vi "Set VI Separate Compiled Code.vi"() -> ()   [LabVIEW 2016]
doc: "A wrapper engine for setting separate compiled code for all VIs in a folder."
uses:
  <vilib>/Utility/error.llb/DialogType.ctl
  SLL Queued State Machine/Queue Driver/Create Queue.vi
  SLL Queued State Machine/Queue Driver/Enqueue an Item to Queue.vi
  SLL Queued State Machine/Queue Driver/Dequeue Queue.vi
  SLL Queued State Machine/Queue Driver/Enqueue N Items.vi
  SLL Queued State Machine/Queue Driver/Flush Queue.vi
  SLL Queued State Machine/Queue Driver/Release Queue.vi
  SLL Queued State Machine/SLL QSM.lvlib
panel:
  out "Progress":i32
  in  "Separate Compiled Code?":bool=TRUE
  out "VI List[]":path[](array[path])
  in  "Folder Path":path
  out "Status":string
  in  "Run":bool
  # "Set VI Separate Compiled Code"
  # "Sets the separate compile code property for the VIs in the folder"
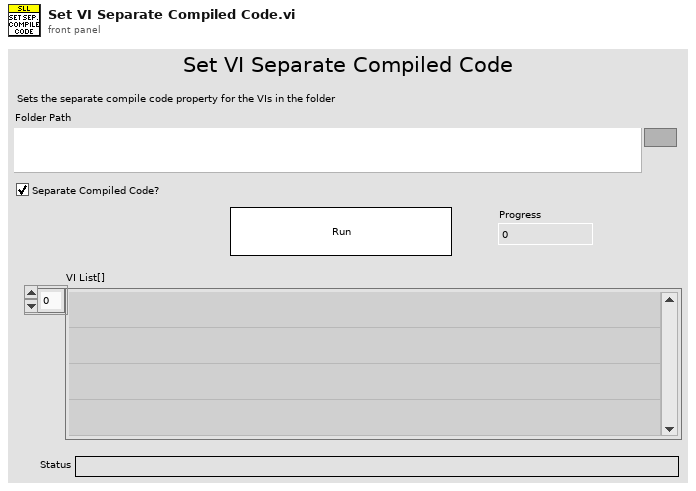
[diagram p1: front panel]
types:
  T1 = typedef "DialogType.ctl" = u16
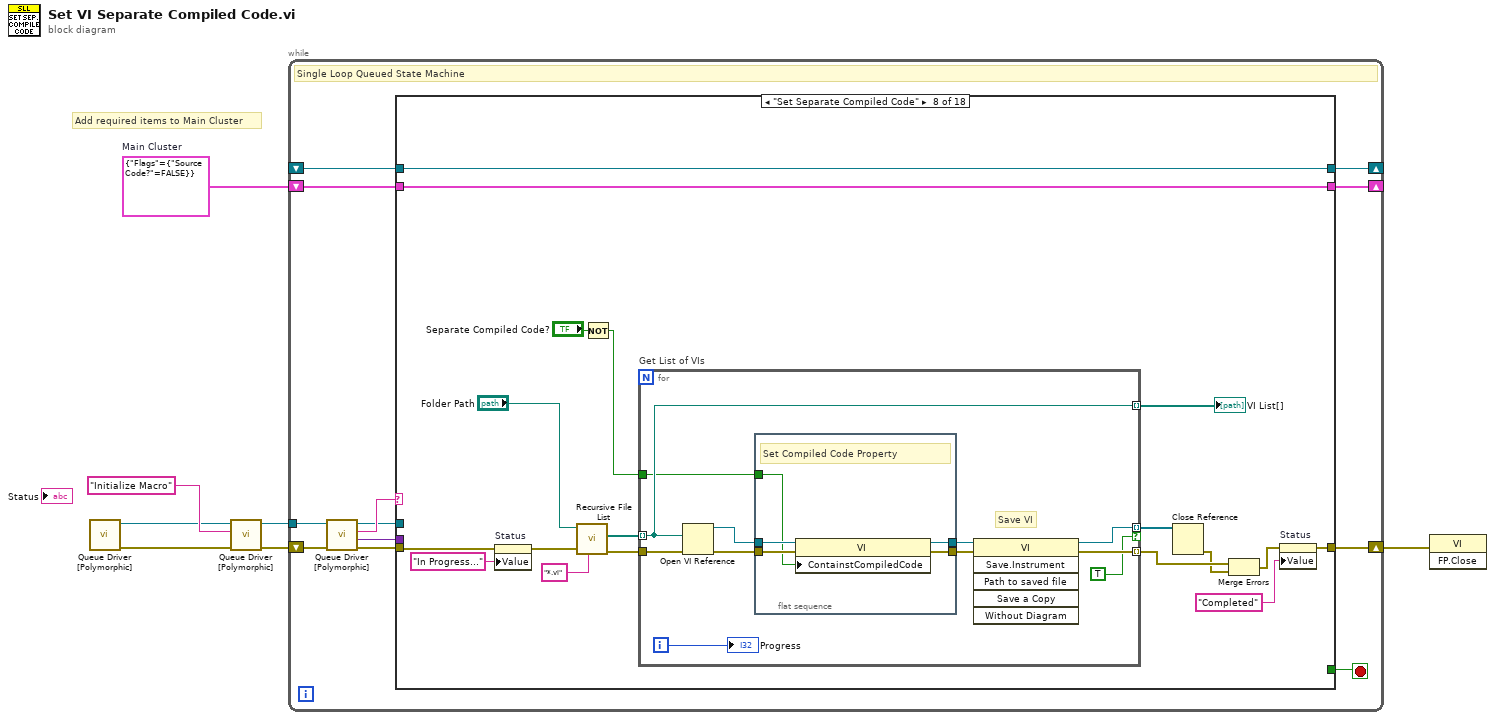
[diagram p0: block diagram]
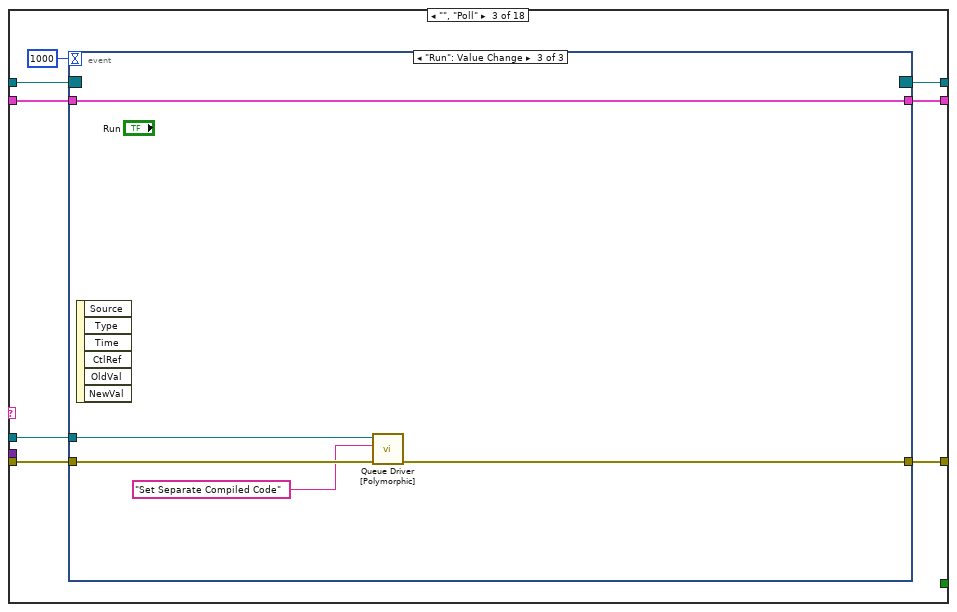
[diagram p4: hidden frame]
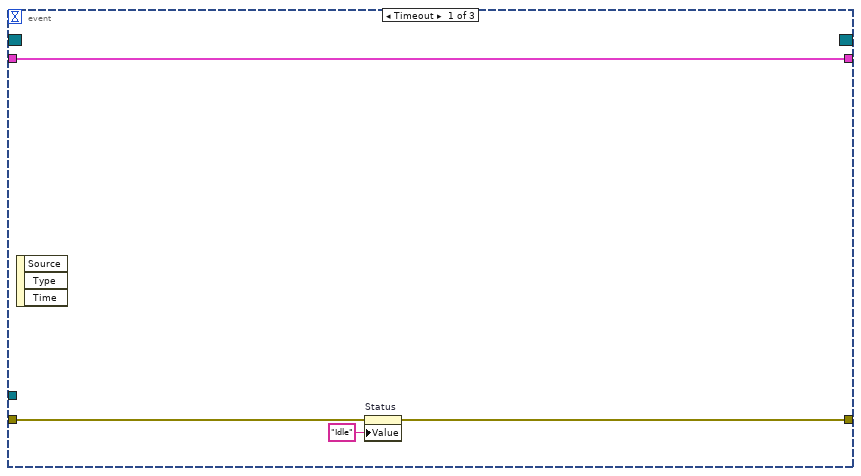
[diagram p5: hidden frame]
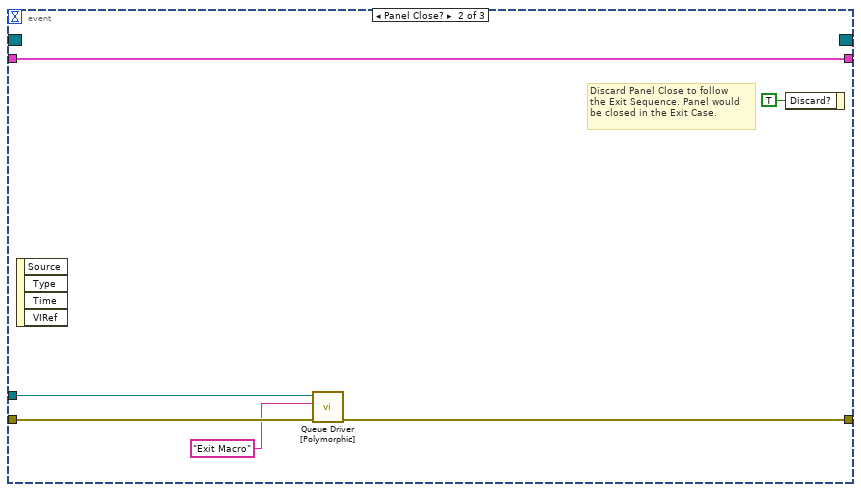
[diagram p6: hidden frame]
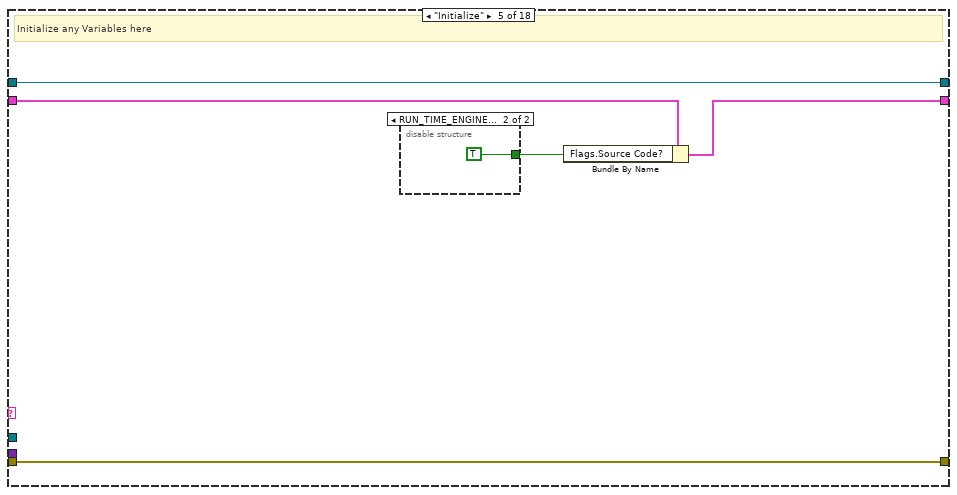
[diagram p8: hidden frame]
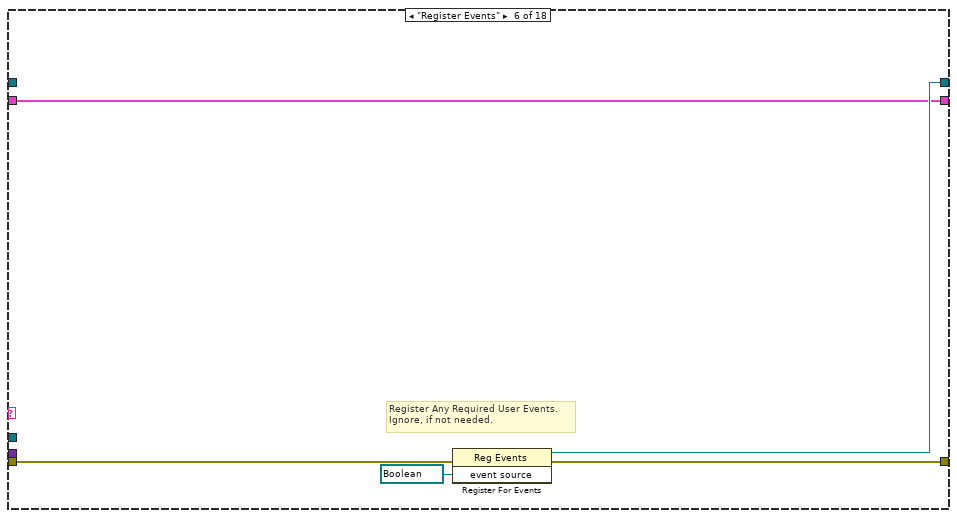
[diagram p10: hidden frame]
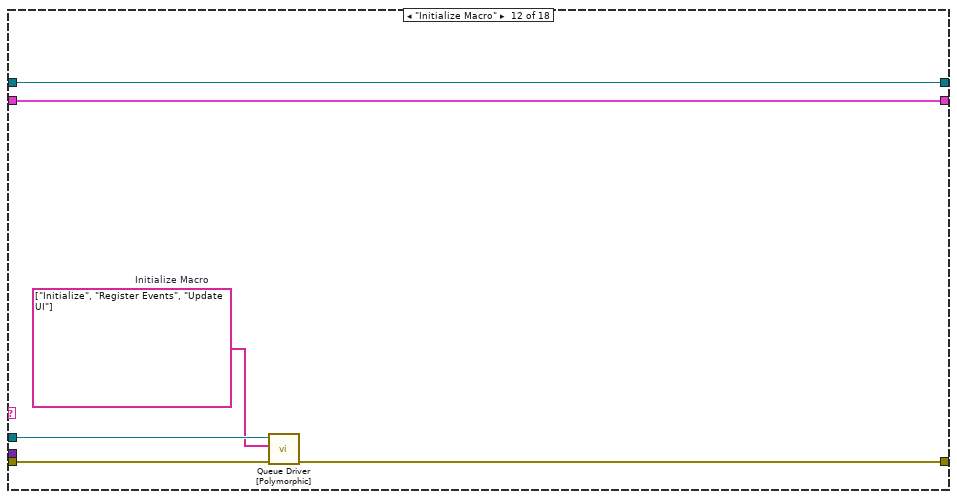
[diagram p15: hidden frame]
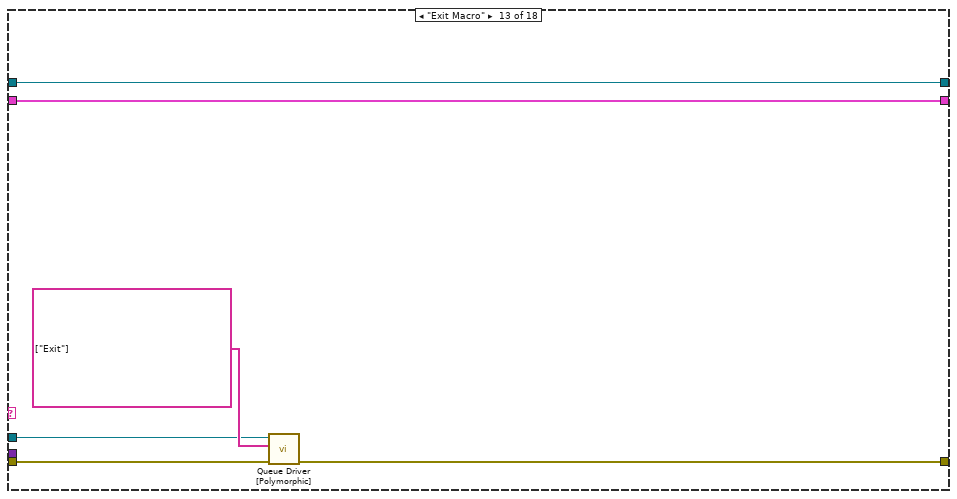
[diagram p16: hidden frame]
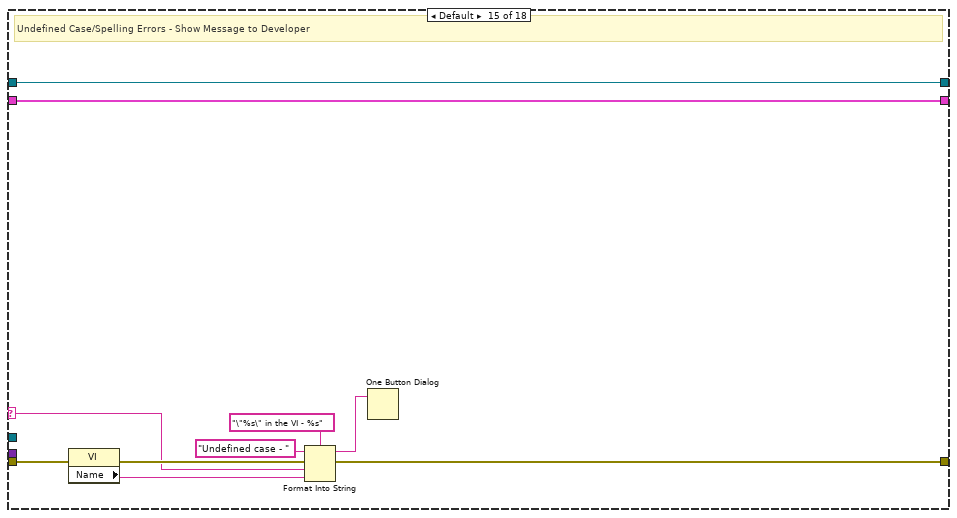
[diagram p18: hidden frame]
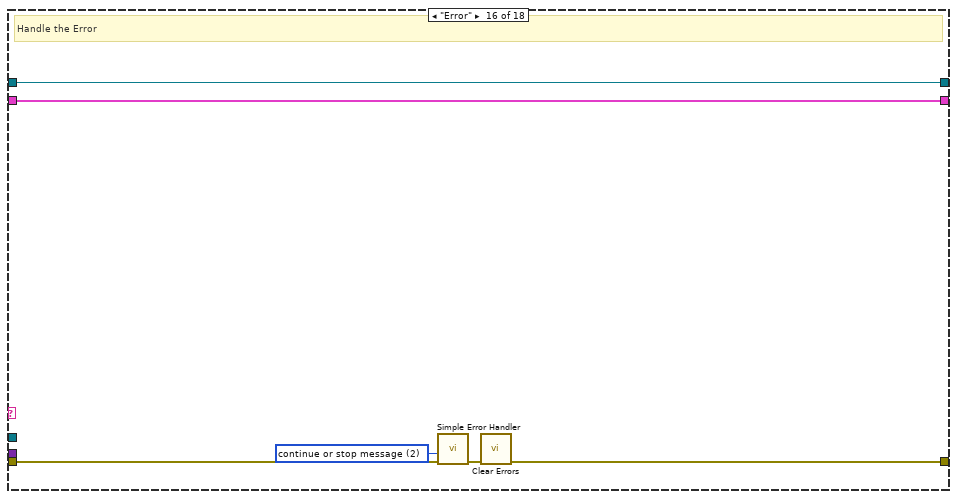
[diagram p19: hidden frame]
diagram:
  w5 = cluster{"Flags":cluster{"Source Code?":bool}} {"Flags"={"Source Code?"=FALSE}}  # Main Cluster
  # "Add required items to Main Cluster"
  n1 = call-poly "Queue Driver [Polymorphic].vi"() -> ("Error Out"=w7:errorcluster, "Queue Ref"=w3:refnum<queue>)  [unwired: 10 in]
  n2 = call-poly "Queue Driver [Polymorphic].vi"("Error In"=w7, "Item to Add"="Initialize Macro", "Queue Ref In"=w3) -> ("Error Out"=w6:errorcluster, "Queue Ref Out"=w2:refnum<queue>)  [unwired: 7 in]
  n3 = while "SLL Queued State Machine" {
    shift-right: [w17] -> w1
    shift-left: w6 -> [w19]
    shift-right: [w15] -> _
    shift-left: _ -> [w14]
    shift-right: [w13] -> _
    shift-left: w5 -> [w12]
    tunnel: w2 -> [w10]
    stop <- w16 stop-if-true
    # "Single Loop Queued State Machine"
    n4 = call-poly "Queue Driver [Polymorphic].vi"("Error In"=w19, "Queue Ref In"=w10) -> ("Error Out"=w18:errorcluster, "Data"=w8:variant, "Dequeue"=w11:string, "Queue Ref Out"=w9:refnum<queue>)  [unwired: 6 in]
    n5 = case "QSM Case Structure" shown="\"Set Separate Compiled Code\"" w11 {
      selector: w11 -> [_ _ _ _ _ _ _ _ _ _ _ _ _ _ w124 _ _ _]
      tunnel: w18 -> [w22 w25 w31 w51 w56 w62 w65 w78 w102 w105 w108 w112 w118 w123 w127 w139 w142 w155]
      tunnel: [w22 w25 w32 w51 w56 w61 w65 w80 w102 w105 w108 w111 w117 w123 w130 w137 w142 w151] -> w17
      tunnel: [_ _ _ _ _ _ _ _ _ _ _ _ _ _ _ _ _ TRUE] -> w16
      tunnel: [w21 w24 w30 w50 w55 w60 w64 w83 w101 w104 w107 w114 w120 w122 w133 w136 w141 w154] -> w15
      tunnel: w14 -> [w21 w24 w29 w50 w55 _ w64 w83 w101 w104 w107 w114 w120 w122 w133 w136 w141 w154]
      tunnel: [w20 w23 w27 w49 w52 w59 w63 w82 w100 w103 w106 w113 w119 w121 w132 w135 w140 w153] -> w13
      tunnel: w12 -> [w20 w23 w28 w49 w53 w59 w63 w82 w100 w103 w106 w113 w119 w121 w132 w135 w140 w153]
      tunnel: w9 -> [_ _ w26 _ _ _ _ _ _ _ _ w110 w115 _ _ _ _ w144]
      tunnel: w8 -> [_ _ _ _ _ _ _ _ _ _ _ _ _ _ _ _ _ _]
      frame "/--------------- Read Me -----------------/" {
        # "General Purpose Queue Based State Machine for Any Use Case (main application, module, pop up message etc)\n\nAdvantages:\n1. No Need to Pass Queue References between Queue Driver VIs.\n2. This template can be safely used in multiple parallel running modules without any issues.\n3. This template can also be safely used even in cases where the VI is configured to be a Clone, where multiple \ninstances of the VI could be executing concurrently.\n\nHow to Use:\n1. Add necessary items to the Main Cluster.\n2. Use the Polymorphic Queue Driver for doing any queue operations. There is no need to pass the queue driver\nreference, as the Queue Driver automatically infers the reference based on the VI instance from which it is called.\n3. Add any required user events in the \"Register Events\" case. Ignore if not needed.\n4. Use \"Sequences\" section for defining any list of state calls, which could be used in multiple places. \nEg: Initialize Sequence, might be needed if we need to any reinitialization."
      }
      frame "/------------------ Poll -------------------/" {
      }
      frame "", "Poll" {
        n6 = event shown="[2] \"Run\": Value Change" {
          selector: w29 -> [_ _ _]
          dyn-events: [_ _ _] -> w30
          timeout: 1000 -> [_ _ _]
          tunnel: [w34 w42 w47] -> w32
          tunnel: w31 -> [w35 w43 w48]
          tunnel: w28 -> [w37 w41 w46]
          tunnel: [w37 w41 w46] -> w27
          tunnel: w26 -> [_ w38 w45]
          event Timeout {
            n7 = event-data() -> ()  [unwired: 1 in, 3 out]
            n8 = property on="Status" class="Str"(error in=w35, "Value"="Idle" ("Status")) -> (error out=w34:errorcluster)  [unwired: 1 in, 1 out]
          }
          event Panel Close? {
            # "Discard Panel Close to follow\nthe Exit Sequence. Panel would\nbe closed in the Exit Case."
            n9 = event-data() -> ()  [unwired: 1 in, 4 out]
            n10 = call-poly "Queue Driver [Polymorphic].vi"("Error In"=w43, "Item to Add"="Exit Macro" ("Enqueue"), "Queue Ref In"=w38) -> ("Error Out"=w42:errorcluster)  [unwired: 7 in, 1 out]
            n11 = event-data("Discard?"=TRUE) -> ()  [unwired: 1 in, 1 out]
          }
          event "Run": Value Change {
            n12 = event-data() -> ()  [unwired: 1 in, 6 out]
            n13 = call-poly "Queue Driver [Polymorphic].vi"("Error In"=w48, "Item to Add"="Set Separate Compiled Code", "Queue Ref In"=w45) -> ("Error Out"=w47:errorcluster)  [unwired: 7 in, 1 out]
          }
        }
      }
      frame "/--------------- Initialize -----------------/" {
      }
      frame "Initialize" {
        # "Initialize any Variables here"
        n14 = disable-structure shown="RUN_TIME_ENGINE==False" {
          disable-tunnel: [_ TRUE] -> w54
          frame condition #0 {
          }
          frame condition #1 (active) {
          }
        }
        n15 = Bundle By Name(cluster=w53, "Flags.Source Code?"=w54) -> (w52:cluster{"Flags":cluster{"Source Code?":bool}})
      }
      frame "Register Events" {
        # "Register Any Required User Events. \nIgnore, if not needed."
        n16 = register-events(error in=w62, refnum<vi> refnum ("event source")) -> (reference out=w60:refnum<event-registration>, error out=w61:errorcluster)  [unwired: 1 in]
      }
      frame "/---------- Custom Case Splitter ----------/" {
      }
      frame "Set Separate Compiled Code" {
        n17 = property on="Status" class="Str"(error in=w78, "Value"="In Progress..." ("Status")) -> (error out=w70:errorcluster)  [unwired: 1 in, 1 out]
        n18 = call <vilib>:"Recursive File List.vi"("pattern"="*.vi", "error in (no error)"=w70, "Folder Path"="Folder Path") -> ("error out"=w74:errorcluster, "All Files in Dir"=w75:path[])  [unwired: 4 in, 3 out]
        n19 = Not(x="Separate Compiled Code?") -> (.not. x?=w71:bool)
        n20 = for "Get List of VIs" {
          tunnel: [w92] -> w77 mode=indexing if=TRUE
          tunnel: w75 -> [w89] mode=indexing
          tunnel: [w89] -> w66 mode=indexing
          tunnel: w74 -> [w91]
          tunnel: [w93] -> w73 mode=indexing
          tunnel: w71 -> [w88]
          i -> [w94]
          # "Save VI"
          n21 = Open VI Reference(vi path=w89, error in (no error)=w91) -> (vi reference=w87:refnum<vi>, error out=w86:errorcluster)  [unwired: 4 in]
          n22 = flat-sequence {
            tunnel: w87 -> [w97]
            tunnel: w86 -> [w99]
            tunnel: [w98] -> w85
            tunnel: [w96] -> w84
            tunnel: w88 -> [w95]
            frame #0 {
              # "Set Compiled Code Property"
              n23 = property class="VI"(reference=w97, error in=w99, "ContainstCompiledCode"=w95) -> (reference out=w96:refnum<vi>, error out=w98:errorcluster)
            }
          }
          n24 = invoke class="VI" method="Save.Instrument"(reference=w84, error in=w85) -> (reference out=w92:refnum<vi>, error out=w93:errorcluster)  [unwired: 4 in, 4 out]
          "Progress" <- w94
        }
        "VI List[]" <- w66
        n25 = Close Reference(reference=w77) -> (error out=w72:errorcluster)  [unwired: 1 in]
        n26 = Merge Errors(w73, w72) -> (w67:errorcluster)
        n27 = property on="Status" class="Str"(error in=w67, "Value"="Completed" ("Status")) -> (error out=w80:errorcluster)  [unwired: 1 in, 1 out]
      }
      frame "/-------------- User Interface --------------/" {
        # "Duplicate this case to create additional case splitters for readability"
      }
      frame "Update UI" {
        # "Update Front Panel Controls in this Case"
      }
      frame "/----------------- Macros -----------------/" {
      }
      frame "Initialize Macro" {
        w109 = string[] ["Initialize", "Register Events", "Update UI"]  # Initialize Macro
        n28 = call-poly "Queue Driver [Polymorphic].vi"("Error In"=w112, "Enqueue N"=w109, "Queue Ref In"=w110) -> ("Error Out"=w111:errorcluster)  [unwired: 7 in, 1 out]
      }
      frame "Exit Macro" {
        n29 = call-poly "Queue Driver [Polymorphic].vi"("Error In"=w118, "Enqueue N"=string[] ["Exit"], "Queue Ref In"=w115) -> ("Error Out"=w117:errorcluster)  [unwired: 7 in, 1 out]
      }
      frame "/-------------- Error Handler--------------/" {
      }
      frame Default {
        # "Undefined Case/Spelling Errors - Show Message to Developer"
        n30 = property class="VI"(error in=w127) -> (error out=w126:errorcluster, "Name"=w125:string)  [unwired: 1 in, 1 out]
        n31 = Format Into String(format string="\"%s\" in the VI - %s" ("message"), initial string="Undefined case - ", error in=w126, w124, w125) -> (resulting string=w128:string, error out=w130:errorcluster)
        n32 = One Button Dialog(message=w128) -> ()  [unwired: 1 in, 1 out]
      }
      frame "Error" {
        w134 = T1 2 items=["no dialog", "OK message", "continue or stop message", "OK message + warnings", "continue/stop + warnings"] ("type of dialog (OK msg:1)")
        # "Handle the Error"
        n33 = call <vilib>:"Simple Error Handler.vi"("type of dialog (OK msg:1)"=w134, "error in (no error)"=w139) -> ("error out"=w138:errorcluster)  [unwired: 3 in, 4 out]
        n34 = call <vilib>:"Clear Errors.vi"("error in (no error)"=w138) -> ("error out"=w137:errorcluster)  [unwired: 5 in, 1 out]
      }
      frame "/------------------- Exit --------------------/" {
      }
      frame "Exit" {
        n35 = call-poly "Queue Driver [Polymorphic].vi"("Error In"=w155, "Queue Ref In"=w144) -> ("Error Out"=w156:errorcluster, "Queue Ref Out"=w143:refnum<queue>)  [unwired: 7 in, 1 out]
        n36 = Unbundle By Name(w153) -> ("Flags.Source Code?"=w146:bool)
        n37 = call-poly "Queue Driver [Polymorphic].vi"("Error In"=w156, "Queue Ref In"=w143) -> ("Error Out"=w152:errorcluster)  [unwired: 9 in]
        n38 = Call Chain() -> (call chain=w150:string[])
        n39 = Array Size(array=w150) -> (size(s)=w149:i32)
        n40 = Equal?(x=w149, y=1) -> (x = y?=w147:bool)
        n41 = And(x=w146, y=w147) -> (x .and. y?=w145:bool)
        n42 = case "Skip Panel Close when in Source\nCode and is the top most caller" shown="True" w145 {
          tunnel: w152 -> [w159 w161]
          tunnel: [w160 w161] -> w151
          frame False {
            # "Close Panel"
            n43 = invoke class="VI" method="FP.Close"() -> (error out=w158:errorcluster)  [unwired: 3 in, 2 out]
            n44 = Merge Errors(w159, w158) -> (w160:errorcluster)
          }
          frame True {
            # "Do Not Close Panel"
          }
        }
      }
    }
  }
  n45 = invoke class="VI" method="FP.Close"(error in=w1) -> ()  [unwired: 2 in, 3 out]
